vi "题目3.vi"() -> ()   [LabVIEW 2017]
panel:
  out "数组":dbl[][](array[numeric])
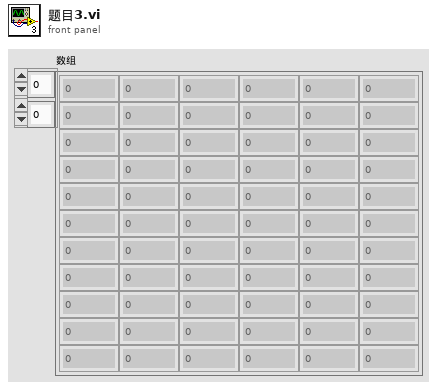
[diagram p1: front panel]
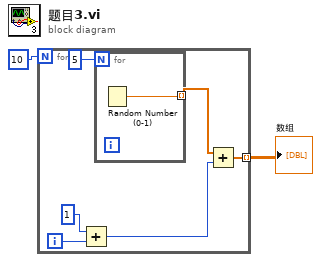
[diagram p0: block diagram]
diagram:
  n1 = for {
    N: 10 -> [_]
    tunnel: [w3] -> w1 mode=indexing
    i -> [w6]
    n2 = Add(x=1, y=w6) -> (x+y=w4:i32)
    n3 = for {
      N: 5 -> [_]
      tunnel: [w9] -> w7 mode=indexing
      n4 = Random Number (0-1)() -> (number: 0 to 1=w9:dbl)
    }
    n5 = Add(x=w7, y=w4) -> (x+y=w3:dbl[])
  }
  "数组" <- w1
